vi "test Swap Data.vi"(8 "error in (no error)":errorcluster, 11 "TestCase in":refnum<class "Data Manipulation Tests.lvclass">) -> (0 "error out":errorcluster, 3 "TestCase out":refnum<class "Data Manipulation Tests.lvclass">)   [LabVIEW 2020, in "Memory Manager Tests.lvlib" / "Data Manipulation Tests.lvclass"]
uses:
  Data Manipulation Tests.lvclass
  Source/Classes/Pointer/Write 1D I32.vi
  Source/Classes/Pointer/Read 1D I32.vi
  <vilib>/addons/_JKI Toolkits/VI Tester/TestCase.llb/TestCase.lvclass
  Source/Classes/Pointer/Pointer.lvclass
  C:/Program Files (x86)/National Instruments/LabVIEW 2020/vi.lib/addons/_JKI Toolkits/VI Tester/TestCase.llb/TestCase.lvclass
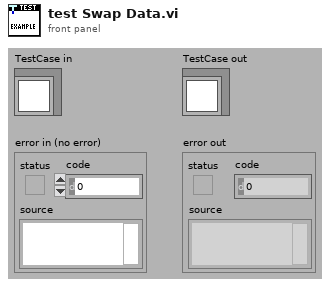
[diagram p1: front panel]
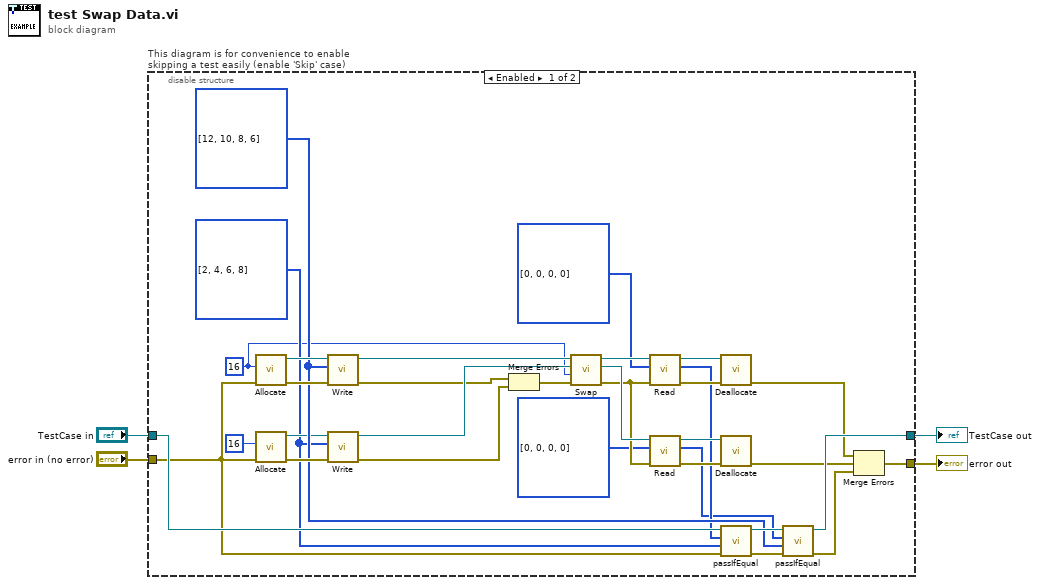
[diagram p0: block diagram]
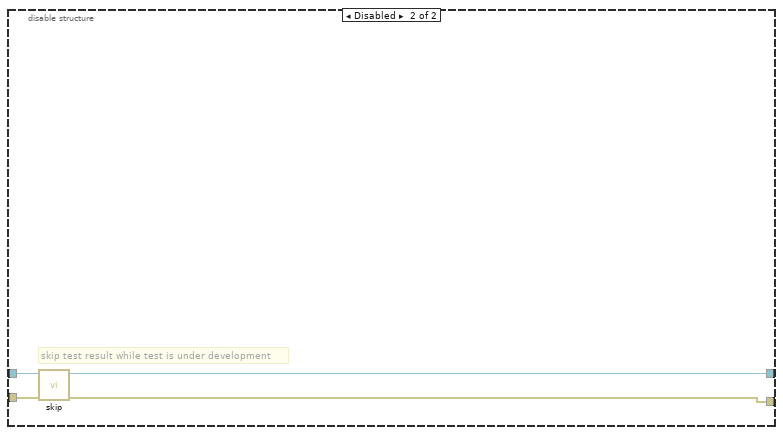
[diagram p2: hidden frame]
diagram:
  n1 = disable-structure "This diagram is for convenience to enable skipping a test easily (enable 'Skip' case)" shown="Enabled" {
    disable-tunnel: "TestCase in" -> [w31 w41]
    disable-tunnel: [w28 w39] -> w1
    disable-tunnel: [w19 w40] -> w3
    disable-tunnel: "error in (no error)" -> [w20 w38]
    frame Enabled {
      w10 = i32[] [2, 4, 6, 8] ("buffer in")
      w12 = i32[] [12, 10, 8, 6] ("buffer in")
      w5 = u64 16 ("count (1)")
      n2 = call "Allocate.vi"("error in (no error)"=w20, "size"=w5) -> ("error out"=w22:errorcluster, "Pointer out"=w36:refnum<class "Pointer.lvclass">)  [unwired: 8 in]
      n3 = call "Allocate.vi"("error in (no error)"=w20, "size"=u64 16 ("count (1)")) -> ("error out"=w26:errorcluster, "Pointer out"=w11:refnum<class "Pointer.lvclass">)  [unwired: 8 in]
      n4 = call-poly "Write.vi"("error in (no error)"=w22, "buffer in"=w12, "Pointer in"=w36) -> ("error out"=w23:errorcluster, "Pointer out"=w35:refnum<class "Pointer.lvclass">)  [unwired: 5 in, 2 out]
      n5 = call-poly "Write.vi"("error in (no error)"=w26, "buffer in"=w10, "Pointer in"=w11) -> ("error out"=w25:errorcluster, "Pointer out"=w34:refnum<class "Pointer.lvclass">)  [unwired: 5 in, 2 out]
      n6 = Merge Errors(w23, w25) -> (w24:errorcluster)
      n7 = call "Swap.vi"("error in (no error)"=w24, "size"=w5, "Pointer y"=w34, "Pointer x"=w35) -> ("error out"=w21:errorcluster, "Pointer y"=w32:refnum<class "Pointer.lvclass">, "Pointer x"=w33:refnum<class "Pointer.lvclass">)  [unwired: 5 in]
      n8 = call-poly "Read.vi"("error in (no error)"=w21, "buffer in"=i32[] [0, 0, 0, 0], "Pointer in"=w33) -> ("error out"=w17:errorcluster, "buffer out"=w8:i32[], "Pointer out"=w15:refnum<class "Pointer.lvclass">)  [unwired: 5 in, 1 out]
      n9 = call-poly "Read.vi"("error in (no error)"=w21, "buffer in"=i32[] [0, 0, 0, 0], "Pointer in"=w32) -> ("error out"=w18:errorcluster, "buffer out"=w6:i32[], "Pointer out"=w16:refnum<class "Pointer.lvclass">)  [unwired: 5 in, 1 out]
      n10 = call "Deallocate.vi"("error in (no error)"=w17, "Pointer"=w15) -> ("error out"=w14:errorcluster)  [unwired: 8 in, 1 out]
      n11 = call "Deallocate.vi"("error in (no error)"=w18, "Pointer"=w16) -> ("error out"=w13:errorcluster)  [unwired: 8 in, 1 out]
      n12 = call-dynamic "passIfEqual.vi"("error in (no error)"=w20, "y"=w10, "x"=w8, "TestCase in"=w31) -> ("error out"=w30:errorcluster, "TestCase out"=w29:refnum<class "Data Manipulation Tests.lvclass">)  [unwired: 6 in]
      n13 = call-dynamic "passIfEqual.vi"("error in (no error)"=w30, "y"=w12, "x"=w6, "TestCase in"=w29) -> ("error out"=w27:errorcluster, "TestCase out"=w28:refnum<class "Data Manipulation Tests.lvclass">)  [unwired: 6 in]
      n14 = Merge Errors(w14, w13, w27) -> (w19:errorcluster)
    }
    frame Disabled {
      # "skip test result while test is under development"
      n15 = call <vilib>:"skip.vi"("error in (no error)"=w38, "TestCase in"=w41) -> ("error out"=w40:errorcluster, "TestCase out"=w39:refnum<class "Data Manipulation Tests.lvclass">)  [unwired: 8 in]
    }
  }
  "error out" <- w3
  "TestCase out" <- w1
